vi "Pot Points.vi"(7 "Potting Surface Type":T1, 8 "error in":errorcluster, 10 "Points":T2[](array[typedef]), 11 "SyringeTool in":refnum<class "SyringeTool Class.lvclass">) -> (0 "error out":errorcluster, 3 "SyringeTool out":refnum<class "SyringeTool Class.lvclass">)   [LabVIEW 2011, in "SyringeTool Class.lvclass"]
uses:
  SyringeTool Class.lvclass
  Utils/Type Definitions/3d Point.ctl
  Vec3d Class/Vec3d Class.lvclass
  Config Manager Class/Type Definitions/Potting Surface Type.ctl
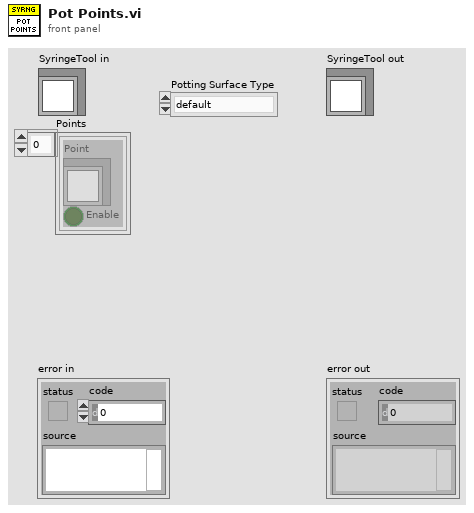
[diagram p1: front panel]
types:
  T1 = typedef "Potting Surface Type.ctl" = enum16{"default", "hdi_edge_pads"}
  T2 = typedef "3d Point.ctl" = cluster{"Point":refnum<class "Vec3d Class.lvclass">, "Enable":bool}
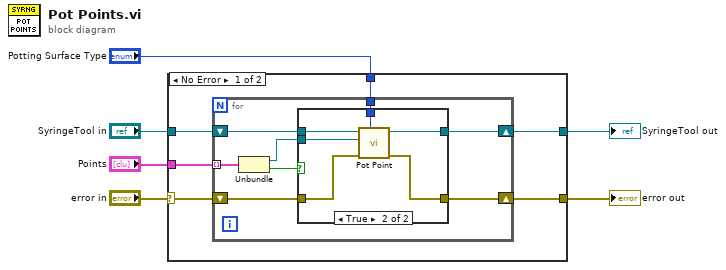
[diagram p0: block diagram]
diagram:
  n1 = case shown="No Error" "error in" {
    selector: "error in" -> [w10 w30]
    tunnel: [w9 w30] -> w5
    tunnel: [w11 w29] -> w3
    tunnel: "SyringeTool in" -> [w12 w29]
    tunnel: "Points" -> [w8 _]
    tunnel: "Potting Surface Type" -> [w7 _]
    frame No Error {
      n2 = for {
        shift-right: [w19] -> w11
        shift-left: w12 -> [w20]
        shift-right: [w17] -> w9
        shift-left: w10 -> [w18]
        tunnel: w8 -> [w16] mode=indexing
        tunnel: w7 -> [w13]
        n3 = Unbundle(w16) -> ("Point"=w14:refnum<class "Vec3d Class.lvclass">, "Enable"=w15:bool)
        n4 = case shown="True" w15 {
          tunnel: w20 -> [w22 w28]
          tunnel: [w22 w27] -> w19
          tunnel: w18 -> [w21 w26]
          tunnel: [w21 w25] -> w17
          tunnel: w14 -> [_ w24]
          tunnel: w13 -> [_ w23]
          frame False {
          }
          frame True {
            n5 = call-dynamic "Pot Point.vi"("Potting Surface Type"=w23, "error in"=w26, "Point"=w24, "SyringeTool in"=w28) -> ("error out"=w25:errorcluster, "SyringeTool out"=w27:refnum<class "SyringeTool Class.lvclass">)  [unwired: 6 in]
          }
        }
      }
    }
    frame Error {
    }
  }
  "error out" <- w5
  "SyringeTool out" <- w3
